vi "FTW-ActorTemplate-RT-TopLevel.vi"   [LabVIEW 2013]
uses:
  src/Instance/FTW-ActorInstance.lvclass
  src/Message/Base/FTW-Message.lvclass
  src/Instance/FTW-ActorInstance.lvclass/FTW-ActorInstance.ctl
  src/JobSequencer/FTW-SEQ-Current.vi
  src/Message/Request/FTW-Message-IncomingRequest.lvclass
  src/Ether/FTW-Ether.lvclass
types:
  T1 = cluster{"Incoming Requests":refnum<event-registration>, "Additional Registration Types":refnum<event-registration>}
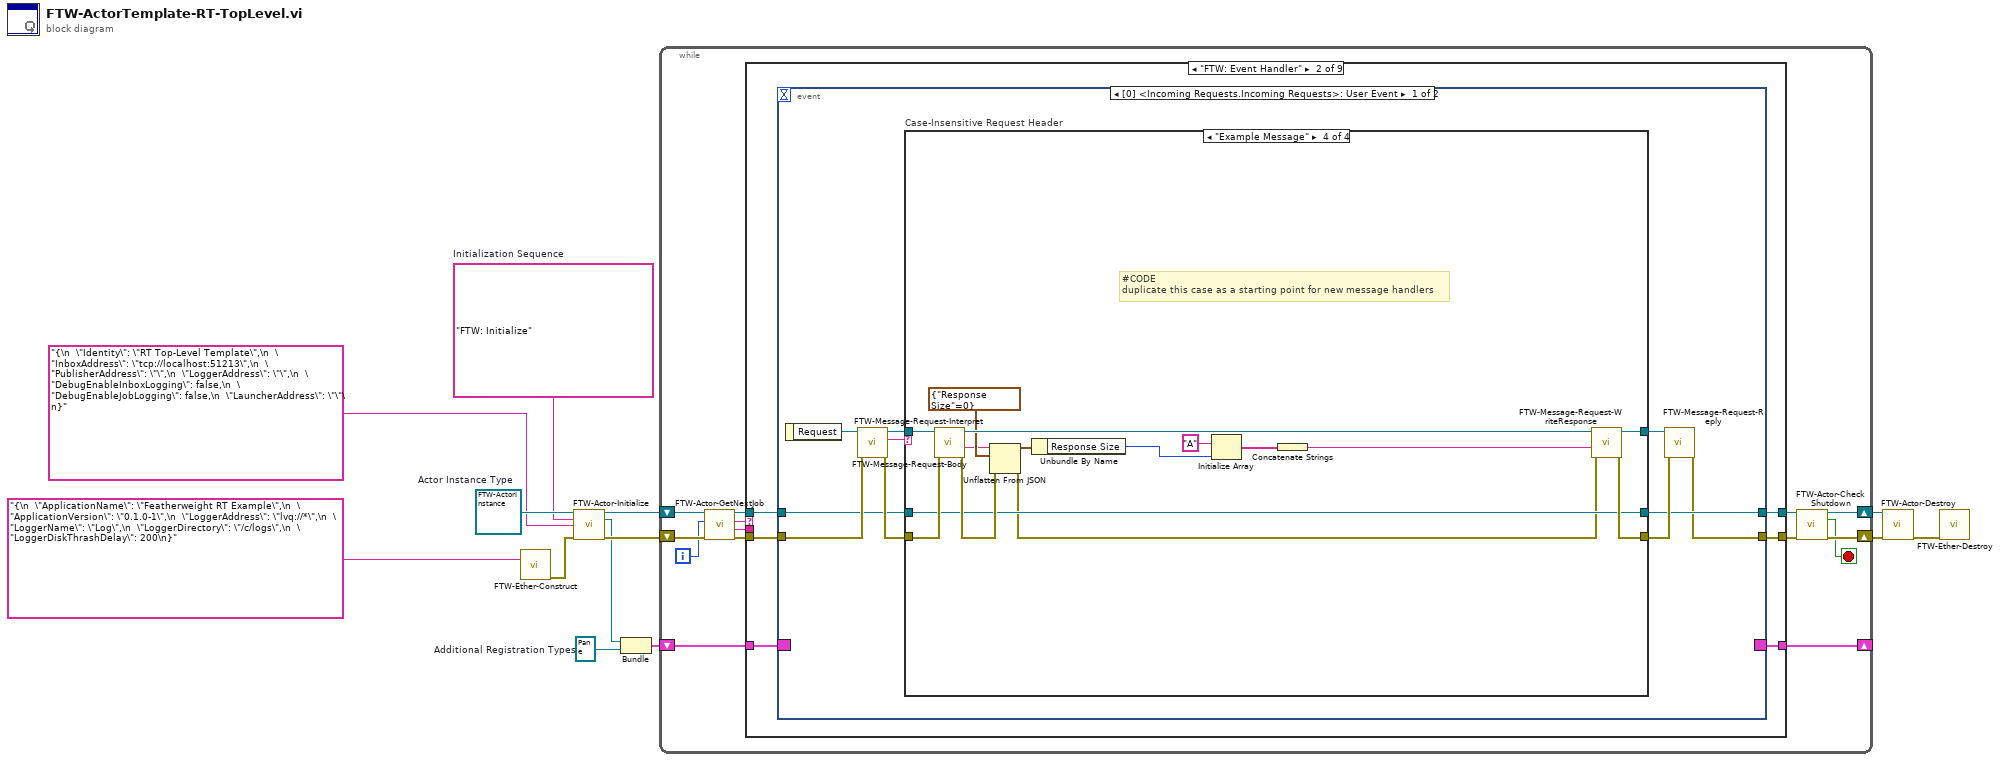
[diagram p0: block diagram]
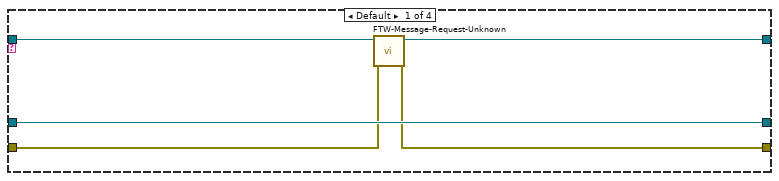
[diagram p3: hidden frame]
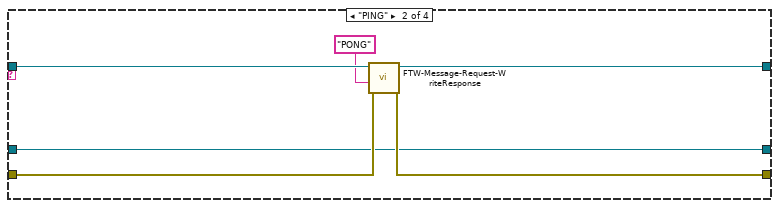
[diagram p4: hidden frame]
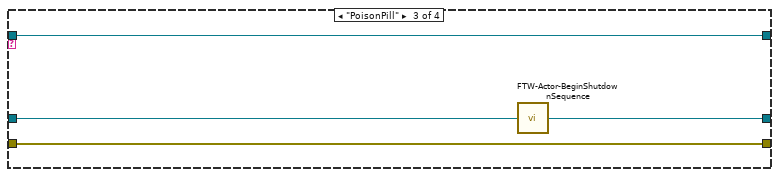
[diagram p5: hidden frame]
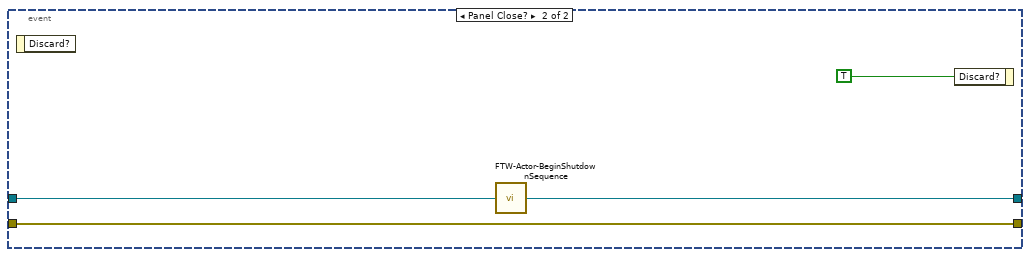
[diagram p6: hidden frame]
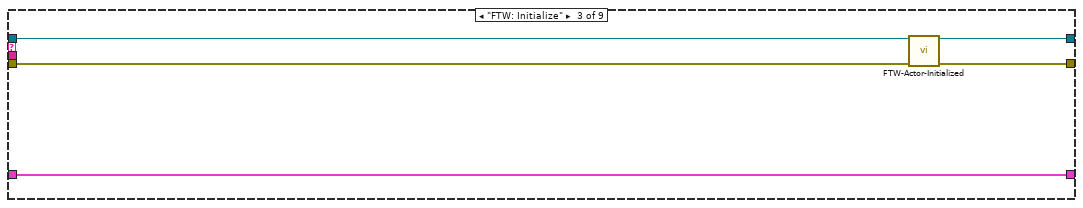
[diagram p7: hidden frame]
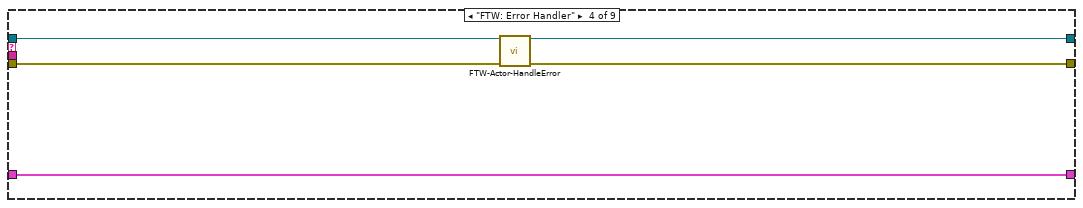
[diagram p8: hidden frame]
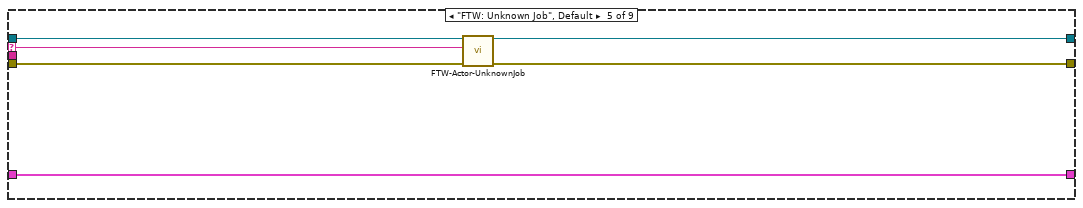
[diagram p9: hidden frame]
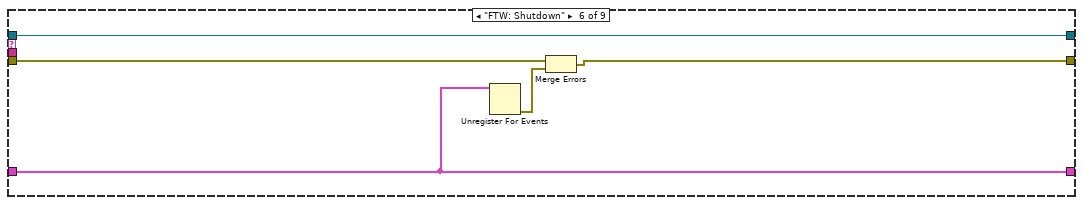
[diagram p10: hidden frame]
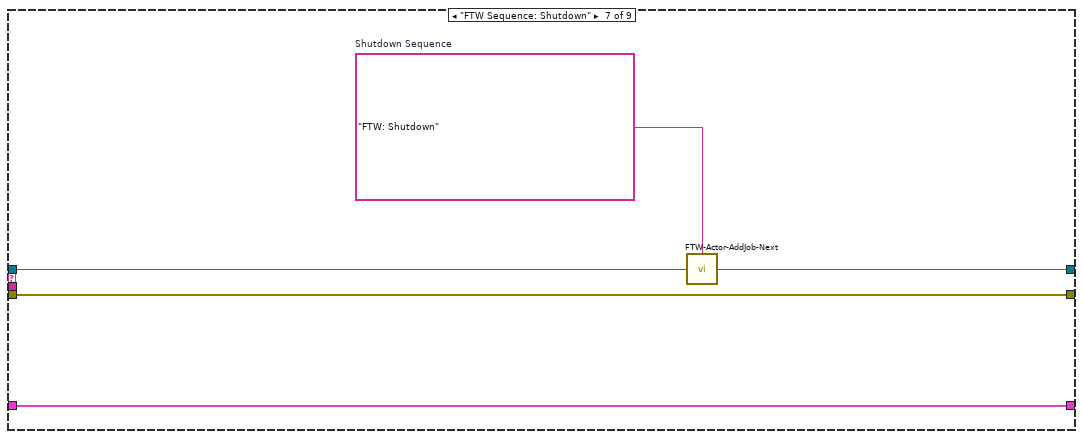
[diagram p11: hidden frame]
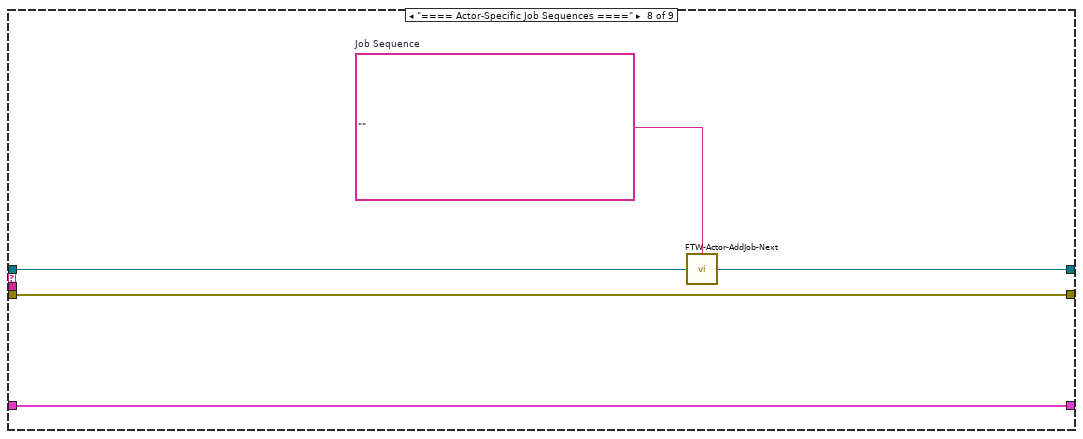
[diagram p12: hidden frame]
diagram:
  w3 = refnum<event-registration> refnum  # Additional Registration Types
  w8 = refnum<class "FTW-ActorInstance.lvclass"> refnum  # Actor Instance Type
  w7 = "FTW: Initialize"  # Initialization Sequence
  n1 = call "FTW-Ether-Construct.vi"("FTW Ether Configuration"="{\n  \"ApplicationName\": \"Featherweight RT Example\",\n  \"ApplicationVersion\": \"0.1.0-1\",\n  \"LoggerAddress\": \"lvq://*\",\n  \"LoggerName\": \"Log\",\n  \"LoggerDirectory\": \"/c/logs\",\n  \"LoggerDiskThrashDelay\": 200\n}") -> ("error out"=w2:errorcluster)  [unwired: 14 in]
  n2 = call-dynamic "FTW-Actor-Initialize.vi"("FTW Actor Instance Type"=w8, "Initialization Job Sequence"=w7, "Actor Instance Configuration"="{\n  \"Identity\": \"RT Top-Level Template\",\n  \"InboxAddress\": \"tcp://localhost:51213\",\n  \"PublisherAddress\": \"\",\n  \"LoggerAddress\": \"\",\n  \"DebugEnableInboxLogging\": false,\n  \"DebugEnableJobLogging\": false,\n  \"LauncherAddress\": \"\"\n}" ("FTW Actor Instance Configuration"), "error in"=w2) -> ("FTW Actor Instance"=w13:refnum<class "FTW-ActorInstance.lvclass">, "Incoming Requests"=w4:refnum<event-registration>, "error out"=w9:errorcluster)  [unwired: 8 in, 1 out]
  n3 = Bundle("Incoming Requests"=w4, "Additional Registration Types"=w3) -> (w6:T1)  [unwired: 1 in]
  n4 = while {
    shift-right: [w17] -> w11
    shift-left: w9 -> [w24]
    shift-right: [w14] -> _
    shift-left: w6 -> [w27]
    shift-right: [w19] -> w12
    shift-left: w13 -> [w26]
    i -> [w15]
    stop <- w16 stop-if-true
    n5 = call "FTW-Actor-GetNextJob.vi"("error in"=w24, "Jobs Performed"=w15, "FTW Actor Instance"=w26) -> ("error out"=w23:errorcluster, "Job Data"=w21:string, "Job Name"=w22:string, "FTW Actor Instance out"=w25:refnum<class "FTW-ActorInstance.lvclass">)  [unwired: 5 in]
    n6 = case shown="\"FTW: Event Handler\"" w22 {
      selector: w22 -> [_ _ _ _ w91 _ _ _ _]
      tunnel: [w29 w36 w81 w86 w94 w100 w105 w110 w114] -> w18
      tunnel: w23 -> [w29 w35 w84 w88 w95 w101 w105 w110 w114]
      tunnel: w27 -> [w30 w31 w85 w90 w96 w97 w106 w111 w113]
      tunnel: [w30 w34 w85 w90 w96 w97 w106 w111 w113] -> w14
      tunnel: w21 -> [_ _ _ _ _ _ _ _ _]
      tunnel: [w28 w33 w82 w87 w92 w98 w103 w108 w112] -> w20
      tunnel: w25 -> [w28 w32 w83 w89 w93 w98 w104 w109 w112]
      frame "==== Featherweight Framework Jobs ====" {
      }
      frame "FTW: Event Handler" {
        n7 = event shown="[0] <Incoming Requests.Incoming Requests>: User Event" {
          selector: w31 -> [_ _]
          dyn-events: [_ _] -> w34
          timeout: _ -> [_ _]
          tunnel: [w38 w79] -> w36
          tunnel: w35 -> [w44 w79]
          tunnel: [w42 w77] -> w33
          tunnel: w32 -> [w41 w78]
          event User Event {
            n8 = event-data() -> ("Request"=w45:refnum<class "FTW-Message-IncomingRequest.lvclass">)  [unwired: 1 in]
            n9 = call "FTW-Message-Request-Interpret.vi"("error in"=w44, "FTW Incoming Request"=w45) -> ("error out"=w46:errorcluster, "Request Header"=w40:string, "FTW Incoming Request out"=w39:refnum<class "FTW-Message-IncomingRequest.lvclass">)  [unwired: 7 in]
            n10 = case "Case-Insensitive Request Header" shown="\"Example Message\"" w40 {
              tunnel: [w49 w55 w60 w73] -> w43
              tunnel: w46 -> [w50 w56 w60 w76]
              tunnel: [w51 w54 w61 w70] -> w42
              tunnel: w41 -> [w51 w54 w59 w70]
              tunnel: w39 -> [w48 w57 w58 w74]
              tunnel: [w47 w53 w58 w71] -> w37
              frame Default {
                n11 = call "FTW-Message-Request-Unknown.vi"("error in"=w50, "FTW Incoming Request"=w48) -> ("error out"=w49:errorcluster, "FTW Incoming Request Out"=w47:refnum<class "FTW-Message-IncomingRequest.lvclass">)  [unwired: 8 in]
              }
              frame "PING" {
                n12 = call "FTW-Message-Request-WriteResponse.vi"("error in"=w56, "Response Body"="PONG" ("Response Header"), "FTW Incoming Request"=w57) -> ("error out"=w55:errorcluster, "FTW Incoming Request out"=w53:refnum<class "FTW-Message-IncomingRequest.lvclass">)  [unwired: 7 in]
              }
              frame "PoisonPill" {
                n13 = call "FTW-Actor-BeginShutdownSequence.vi"("FTW Actor Instance"=w59) -> ("FTW Actor Instance out"=w61:refnum<class "FTW-ActorInstance.lvclass">)  [unwired: 3 in]
              }
              frame "Example Message" {
                # "#CODE\nduplicate this case as a starting point for new message handlers"
                n14 = call "FTW-Message-Request-Body.vi"("error in"=w76, "FTW Incoming Request"=w74) -> ("error out"=w75:errorcluster, "Request Body"=w67:string, "FTW Incoming Request out"=w72:refnum<class "FTW-Message-IncomingRequest.lvclass">)  [unwired: 7 in]
                n15 = Unflatten From JSON(JSON string=w67, type and defaults=cluster{"Response Size":i32} {"Response Size"=0}, error in (no error)=w75) -> (value=w66:cluster{"Response Size":i32}, error out=w69:errorcluster)  [unwired: 4 in]
                n16 = Unbundle By Name(w66) -> ("Response Size"=w65:i32)
                n17 = Initialize Array("A", w65) -> (w63:string[])
                n18 = Concatenate Strings(w63) -> (w62:string)
                n19 = call "FTW-Message-Request-WriteResponse.vi"("error in"=w69, "Response Body"=w62, "FTW Incoming Request"=w72) -> ("error out"=w73:errorcluster, "FTW Incoming Request out"=w71:refnum<class "FTW-Message-IncomingRequest.lvclass">)  [unwired: 7 in]
              }
            }
            n20 = call "FTW-Message-Request-Reply.vi"("error in"=w43, "FTW Incoming Request"=w37) -> ("error out"=w38:errorcluster)  [unwired: 8 in, 1 out]
          }
          event Panel Close? {
            n21 = event-data() -> ()  [unwired: 1 in, 1 out]
            n22 = call "FTW-Actor-BeginShutdownSequence.vi"("FTW Actor Instance"=w78) -> ("FTW Actor Instance out"=w77:refnum<class "FTW-ActorInstance.lvclass">)  [unwired: 3 in]
            n23 = event-data("Discard?"=TRUE) -> ()  [unwired: 1 in, 1 out]
          }
        }
      }
      frame "FTW: Initialize" {
        n24 = call-dynamic "FTW-Actor-Initialized.vi"("FTW Actor Instance"=w83, "error in"=w84) -> ("FTW Actor Instance out"=w82:refnum<class "FTW-ActorInstance.lvclass">, "error out"=w81:errorcluster)  [unwired: 12 in]
      }
      frame "FTW: Error Handler" {
        n25 = call-dynamic "FTW-Actor-HandleError.vi"("FTW Actor Instance"=w89, "error in"=w88) -> ("FTW Actor Instance out"=w87:refnum<class "FTW-ActorInstance.lvclass">, "error out"=w86:errorcluster)  [unwired: 11 in, 1 out]
      }
      frame "FTW: Unknown Job", Default {
        n26 = call-dynamic "FTW-Actor-UnknownJob.vi"("FTW Actor Instance"=w93, "Unknown Job"=w91, "error in"=w95) -> ("FTW Actor Instance out"=w92:refnum<class "FTW-ActorInstance.lvclass">, "error out"=w94:errorcluster)  [unwired: 11 in]
      }
      frame "FTW: Shutdown" {
        n27 = Unregister For Events(event registration refnum=w97) -> (error out=w99:errorcluster)  [unwired: 1 in]
        n28 = Merge Errors(w101, w99) -> (w100:errorcluster)
      }
      frame "FTW Sequence: Shutdown" {
        w102 = "FTW: Shutdown"  # Shutdown Sequence
        n29 = call "FTW-Actor-AddJob-Next.vi"("Add Next in Job Queue"=w102, "FTW Actor Instance"=w104) -> ("FTW Actor Instance out"=w103:refnum<class "FTW-ActorInstance.lvclass">)  [unwired: 2 in]
      }
      frame "==== Actor-Specific Job Sequences ====" {
        w107 = ""  # Job Sequence
        n30 = call "FTW-Actor-AddJob-Next.vi"("Add Next in Job Queue"=w107, "FTW Actor Instance"=w109) -> ("FTW Actor Instance out"=w108:refnum<class "FTW-ActorInstance.lvclass">)  [unwired: 2 in]
      }
      frame "==== Actor-Specific Jobs ====" {
      }
    }
    n31 = call "FTW-Actor-CheckShutdown.vi"("FTW Actor Instance"=w20, "error in"=w18) -> ("FTW Actor Instance out"=w19:refnum<class "FTW-ActorInstance.lvclass">, "Shutdown?"=w16:bool, "error out"=w17:errorcluster)  [unwired: 11 in]
  }
  n32 = call-dynamic "FTW-Actor-Destroy.vi"("FTW Actor Instance"=w12, "error in"=w11) -> ("error out"=w10:errorcluster)  [unwired: 13 in]
  n33 = call "FTW-Ether-Destroy.vi"("error in"=w10) -> ()  [unwired: 14 in, 1 out]
